vi "CreateDebugMessage.vi"(7 "Relationship type":T1=enum."None", 9 "Path":path, 11 "Message":string) -> (3 "Debug message":string)   [LabVIEW 2020, in "DependencyInspection.lvlib" / "CDebugInfo.lvclass"]
uses:
  CDebugInfo.lvclass
  obj/Addons/LabVIEWObjectInterfaces.lvlibp/LabVIEWObjectInterfaces/ILabVIEWItem/RelationshipType.ctl
  obj/Addons/LabVIEWObjectInterfaces.lvlibp/LabVIEWObjectInterfaces/ILabVIEWItem/ILabVIEWItem.lvclass
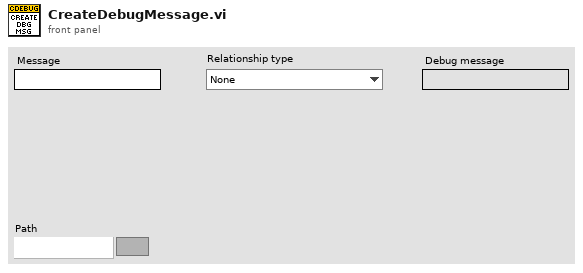
[diagram p1: front panel]
types:
  T1 = typedef "LabVIEWObjectInterfaces.lvlibp/ILabVIEWItem.lvclass/RelationshipType.ctl" = enum16{"Contained", "Dependency", "Parent", "Same item", "Related", "None"}
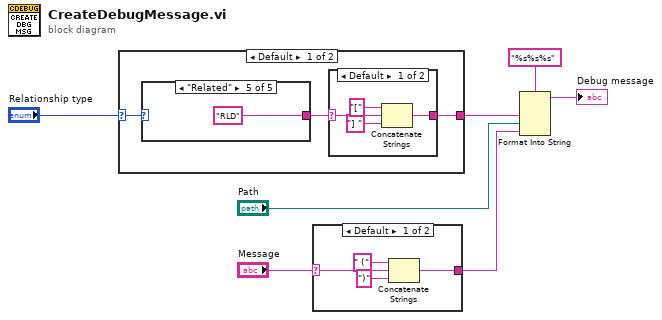
[diagram p0: block diagram]
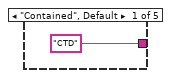
[diagram p2: hidden frame]
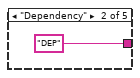
[diagram p3: hidden frame]
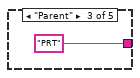
[diagram p4: hidden frame]
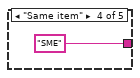
[diagram p5: hidden frame]
diagram:
  n1 = case shown="Default" "Relationship type" {
    selector: "Relationship type" -> [w9 _]
    tunnel: [w10 _] -> w2
    frame Default {
      n2 = case shown="\"Related\"" w9 {
        tunnel: ["CTD" "DEP" "PRT" "SME" "RLD"] -> w8
        frame "Contained", Default {
        }
        frame "Dependency" {
        }
        frame "Parent" {
        }
        frame "Same item" {
        }
        frame "Related" {
        }
      }
      n3 = case shown="Default" w8 {
        selector: w8 -> [w19 w20]
        tunnel: [w18 w20] -> w10
        frame Default {
          n4 = Concatenate Strings("[" ("string"), w19, "] " ("string")) -> (w18:string)
        }
        frame "" {
        }
      }
    }
    frame "None" {
    }
  }
  n5 = case shown="Default" "Message" {
    selector: "Message" -> [w24 w25]
    tunnel: [w23 w25] -> w3
    frame Default {
      n6 = Concatenate Strings(" (" ("string"), w24, ")" ("string")) -> (w23:string)
    }
    frame "" {
    }
  }
  n7 = Format Into String(format string="%s%s%s", w2, "Path", w3) -> (resulting string=→"Debug message":string)  [unwired: 2 in, 1 out]
